vi "Get Handler by Name.vi"(8 "error in (no error)":errorcluster, 10 "Handler Name":string, 11 "Logger in":refnum<class "Logger.lvclass">) -> (0 "error out":errorcluster, 2 "Handler":refnum<class "Handler.lvclass">, 3 "Logger out":refnum<class "Logger.lvclass">)   [LabVIEW 2017, in "Error Log.lvlib" / "Logger.lvclass"]
doc: "Returns the handler with the specified <b>Name</b>.\nIf name was not found, returns a basis handler without functionality and the error \"5030 - Item not found\" is returned."
uses:
  Logger.lvclass
  Handler/Handler.lvclass
  Logger.lvclass/Logger.ctl
  Get Handlers.vi
  Get Handler Names.vi
  <vilib>/Utility/error.llb/Error Cluster From Error Code.vi
  <vilib>/ErrorRing/Error Ring.xnode
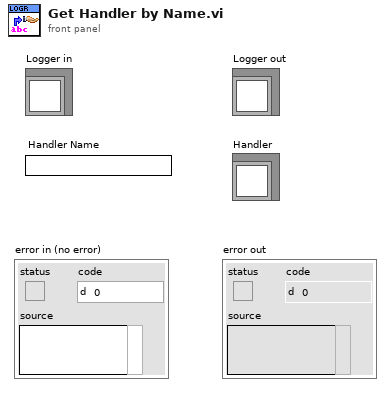
[diagram p1: front panel]
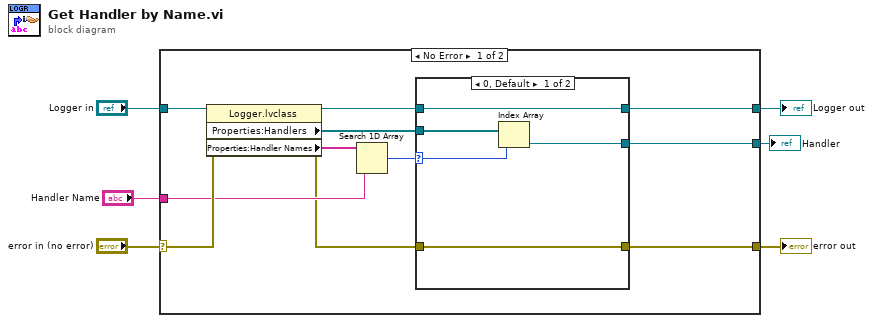
[diagram p0: block diagram]
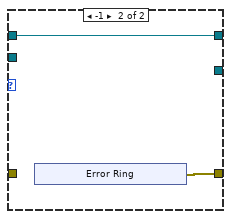
[diagram p2: hidden frame]
diagram:
  n1 = case shown="No Error" "error in (no error)" {
    selector: "error in (no error)" -> [w15 w31]
    tunnel: [w9 w31] -> w5
    tunnel: [w11 w30] -> w3
    tunnel: "Logger in" -> [w16 w30]
    tunnel: "Handler Name" -> [w14 _]
    tunnel: [w7 _] -> w1
    frame No Error {
      n2 = property class="Logger.lvclass"(reference=w16, error in=w15) -> (reference out=w12:refnum<class "Logger.lvclass">, error out=w10:errorcluster, "Properties:Handlers"=w8:refnum<class "Handler.lvclass">[], "Properties:Handler Names"=w17:string[])
      n3 = Search 1D Array(1D array=w17, element=w14) -> (index of element=w13:i32)  [unwired: 1 in]
      n4 = case shown="0, Default" w13 {
        selector: w13 -> [w20 _]
        tunnel: w12 -> [w22 w24]
        tunnel: [w22 w24] -> w11
        tunnel: w10 -> [w18 _]
        tunnel: [w18 w23] -> w9
        tunnel: w8 -> [w21 _]
        tunnel: [w19 _] -> w7
        frame 0, Default {
          n5 = Index Array(array=w21, index=w20) -> (element=w19:refnum<class "Handler.lvclass">)
        }
        frame -1 {
          n6 = xnode "Error Ring"() -> ("error out"=w23:errorcluster)
        }
      }
    }
    frame Error {
    }
  }
  "error out" <- w5
  "Logger out" <- w3
  "Handler" <- w1
